vi "stage_get_position.vi"(8 "error in (no error)":errorcluster, 10 "Stage Name":string, 11 "mcl_piezo in":refnum<class "mcl_piezo.lvclass">) -> (0 "error out":errorcluster, 2 "Position":dbl, 3 "mcl_piezo out":refnum<class "mcl_piezo.lvclass">)   [LabVIEW 2015, in "mcl_piezo.lvclass"]
uses:
  mcl_piezo.lvclass
  mcl_piezo.lvclass/mcl_piezo.ctl
  Madlib.dll
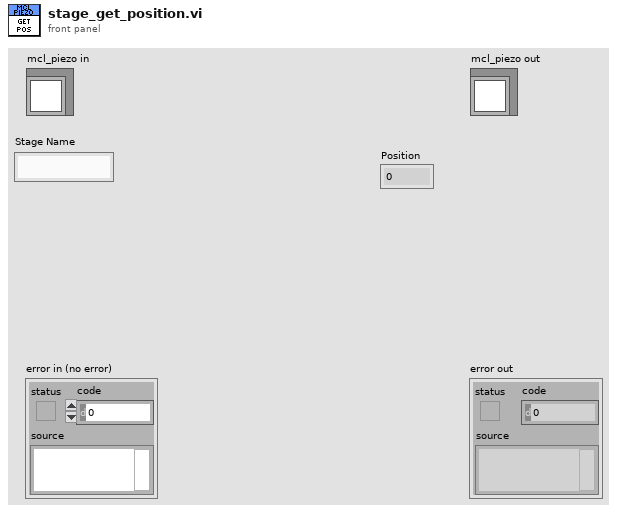
[diagram p1: front panel]
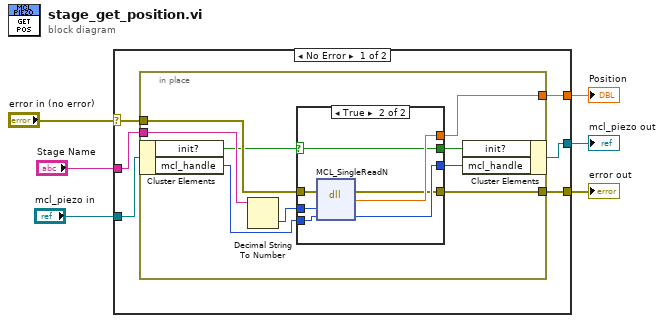
[diagram p0: block diagram]
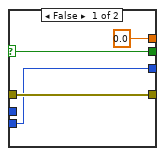
[diagram p2: hidden frame]
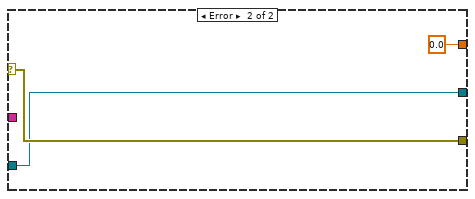
[diagram p3: hidden frame]
diagram:
  n1 = case shown="No Error" "error in (no error)" {
    selector: "error in (no error)" -> [w9 w35]
    tunnel: "Stage Name" -> [w12 _]
    tunnel: "mcl_piezo in" -> [w11 w33]
    tunnel: [w10 0.0] -> w4
    tunnel: [w8 w35] -> w2
    tunnel: [w7 w33] -> w1
    frame No Error {
      n2 = in-place {
        in-place-border: w12 -> [w21]
        in-place-border: [w17] -> w10
        in-place-border: w9 -> [w16]
        in-place-border: [w15] -> w8
        n3 = in-place-cluster #1(w11) -> ("init?"=w14:bool, "mcl_handle"=w19:i32)
        n4 = Decimal String To Number(string=w21) -> (number=w20:i32)  [unwired: 2 in, 1 out]
        n5 = case shown="True" w14 {
          selector: w14 -> [w23 w26]
          tunnel: w20 -> [_ w32]
          tunnel: w19 -> [w22 w31]
          tunnel: [w22 w30] -> w18
          tunnel: [0.0 w29] -> w17
          tunnel: w16 -> [w25 w28]
          tunnel: [w25 w27] -> w15
          tunnel: [w23 w26] -> w13
          frame False {
          }
          frame True {
            n6 = dll-call lib="C:/Users/MX-Microscope/Documents/LabVIEW Data/lvoop_campus_2018/Stage Class/MCL_3d200/MADLib.dll" fn="MCL_SingleReadN"(error in=w28, "axis"=w32, "handle"=w31) -> (error out=w27:errorcluster, w29:dbl, "handle"=w30:i32)  [unwired: 3 in, 1 out]
          }
        }
        n7 = in-place-cluster #1("init?"=w13, "mcl_handle"=w18) -> (w7:refnum<class "mcl_piezo.lvclass">)
      }
    }
    frame Error {
    }
  }
  "error out" <- w2
  "mcl_piezo out" <- w1
  "Position" <- w4
